vi "Read_group_ch.vi"(10 "UnitType":T1(ring)=enum."Power Rider 12") -> (2 "Array":T2(array[cluster]))   [LabVIEW 2017]
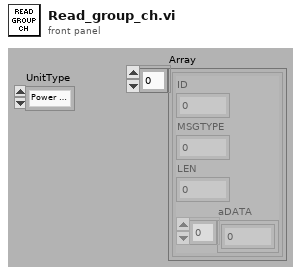
[diagram p1: front panel]
types:
  T1 = enum16{"Single SCB", "Power Rider", "Power Rider&Next10", "HATAL", "DAPH", "Indefinite", "Power Rider 12"}
  T2 = cluster{"ID":u32, "MSGTYPE":u8, "LEN":u8, "aDATA":u8[]}[]
  T3 = cluster{"ID":u32, "MSGTYPE":u8, "LEN":u8, "aDATA":u8[]}
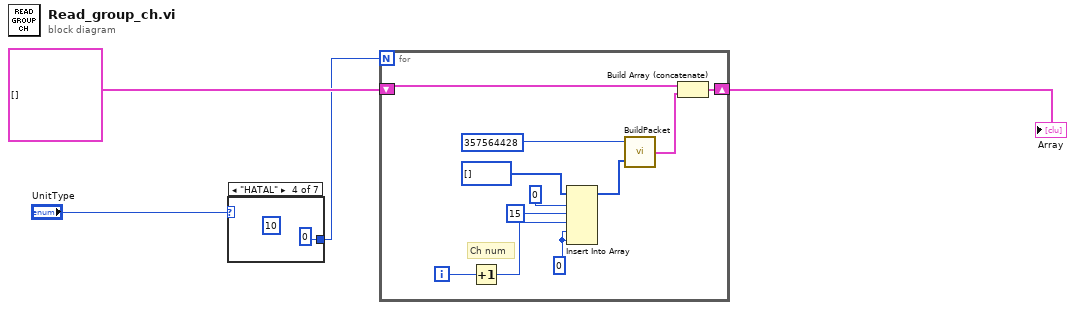
[diagram p0: block diagram]
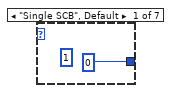
[diagram p2: hidden frame]
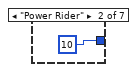
[diagram p3: hidden frame]
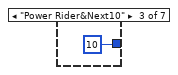
[diagram p4: hidden frame]
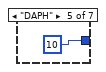
[diagram p5: hidden frame]
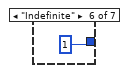
[diagram p6: hidden frame]
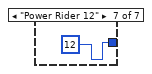
[diagram p7: hidden frame]
diagram:
  n1 = case shown="\"HATAL\"" "UnitType" {
    tunnel: [0 ("Ch_num") 10 ("Ch_num") 10 ("Ch_num") 0 ("Ch_num") 10 ("Ch_num") 1 ("Ch_num") 12 ("Ch_num")] -> w1
    frame "Single SCB", Default {
      (unwired) 1 ("Ch_num")
    }
    frame "Power Rider" {
    }
    frame "Power Rider&Next10" {
    }
    frame "HATAL" {
      (unwired) 10 ("Ch_num")
    }
    frame "DAPH" {
    }
    frame "Indefinite" {
    }
    frame "Power Rider 12" {
    }
  }
  n2 = for {
    N: w1 -> [_]
    shift-right: [w21] -> w3
    shift-left: T2 [] ("Array") -> [w22]
    i -> [w13]
    w15 = u8 0 ("new element/subarray")
    # "Ch num"
    n3 = Increment(x=w13) -> (x+1=w12:i32)
    n4 = Insert Into Array(array=u8[] [] ("Data 2"), index=0, new element #1=u8 15 ("new element/subarray"), new element #2=w12, new element #3=w15, new element #4=w15) -> (w17:u8[])
    n5 = call "BuildPacket.vi"("Data"=w17, "TxID"=u32 357564428) -> ("MsgTX 2"=w19:T3)
    n6 = Build Array (concatenate)(w22, w19) -> (w21:T2)
  }
  "Array" <- w3
